vi "GetPresetSettings.vi"(5 "error in (no error)":errorcluster, 8 "VISA resource name":refnum<visa-resource-name>) -> (0 "error out":errorcluster, 1 "Current":dbl, 2 "Voltage":dbl, 3 "VISA resource name out":refnum<visa-resource-name>, 4 "Preset":dbl)   [LabVIEW 2019, in "9103Series.lvlib"]
uses:
  <instrlib>/9103Series/9103Series.lvlib
panel:
  out "ok?":string
  out "Raw Data":string
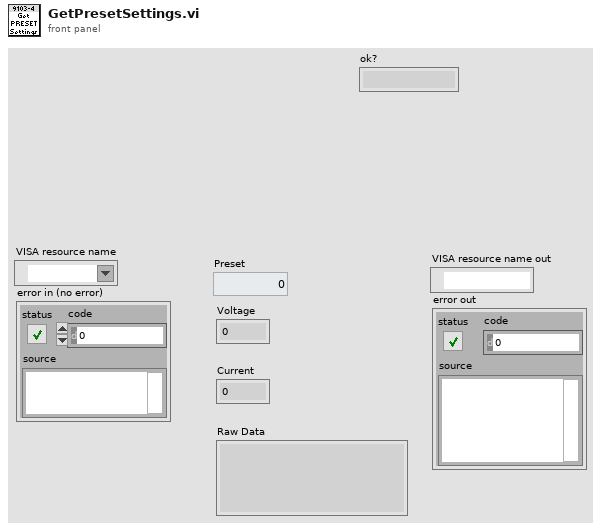
[diagram p1: front panel]
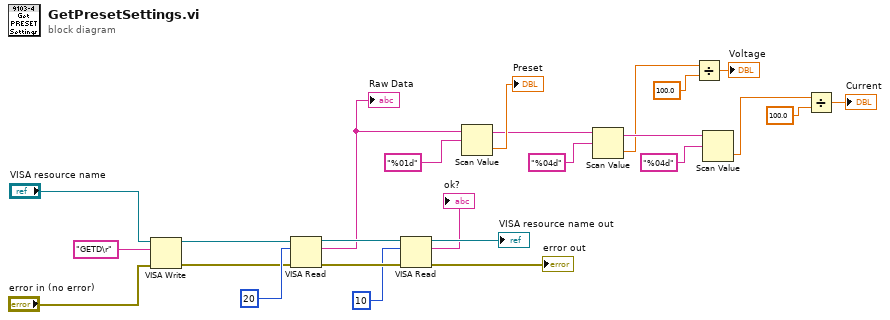
[diagram p0: block diagram]
diagram:
  n1 = VISA Write(VISA resource name="VISA resource name", write buffer="GETD\r", error in (no error)="error in (no error)") -> (VISA resource name out=w21:refnum<visa-resource-name>, error out=w20:errorcluster)  [unwired: 1 out]
  n2 = VISA Read(VISA resource name=w21, byte count=u32 20, error in (no error)=w20) -> (VISA resource name out=w19:refnum<visa-resource-name>, read buffer=w1:string, error out=w18:errorcluster)  [unwired: 1 out]
  "Raw Data" <- w1
  n3 = VISA Read(VISA resource name=w19, byte count=u32 10, error in (no error)=w18) -> (VISA resource name out=→"VISA resource name out":refnum<visa-resource-name>, read buffer=→"ok?":string, error out=→"error out":errorcluster)  [unwired: 1 out]
  n4 = Scan Value(string=w1, format string="%01d") -> (output string=w2:string, value=→"Preset":dbl)  [unwired: 1 in]
  n5 = Scan Value(string=w2, format string="%04d") -> (output string=w11:string, value=w6:dbl)  [unwired: 1 in]
  n6 = Divide(x=w6, y=100.0) -> (x/y=→"Voltage":dbl)
  n7 = Scan Value(string=w11, format string="%04d") -> (value=w9:dbl)  [unwired: 1 in, 1 out]
  n8 = Divide(x=w9, y=100.0) -> (x/y=→"Current":dbl)
